vi "CalcCurrentThreshold.vi"(8 "Target Decimal Output":u8=1, 10 "Current Threshold":dbl=1000.0 format="%#_13g", 11 "Current of Output Pins":dbl[](array[numeric])) -> (0 "Threshold":dbl=1000.0 format="%#_13g", 3 "Target binary output":bool[](array[boolean]))   [LabVIEW 2018]
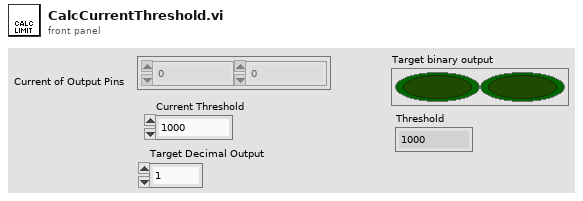
[diagram p1: front panel]
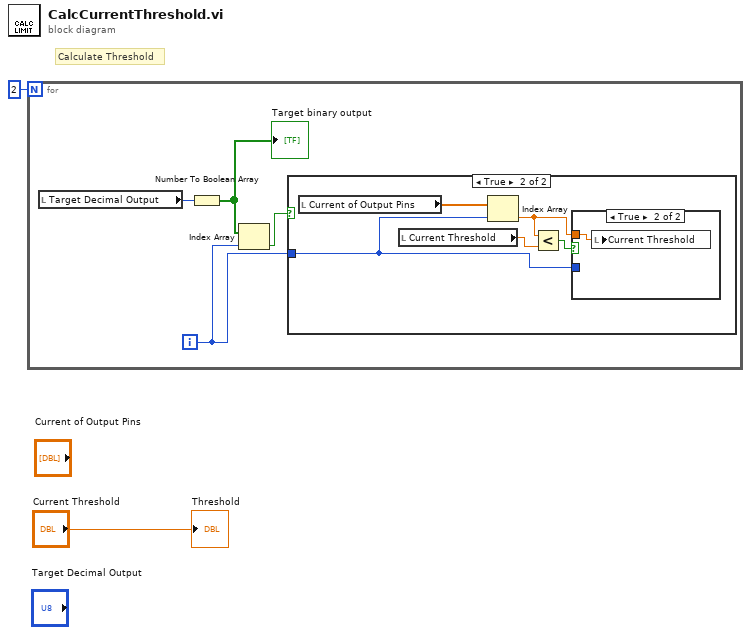
[diagram p0: block diagram]
diagram:
  # "Calculate Threshold"
  n1 = for {
    N: 2 -> [_]
    i -> [w4]
    n2 = local read "Target Decimal Output"() -> (w6:u8)
    n3 = Number To Boolean Array(number=w6) -> (Boolean array=w3:bool[])
    "Target binary output" <- w3
    n4 = Index Array(array=w3, index=w4) -> (element=w5:bool)
    n5 = case shown="True" w5 {
      tunnel: w4 -> [_ w11]
      frame False {
      }
      frame True {
        n6 = local read "Current of Output Pins"() -> (w9:dbl[])
        n7 = local read "Current Threshold"() -> (w7:dbl)
        n8 = Index Array(array=w9, index=w11) -> (element=w8:dbl)
        n9 = Less?(x=w8, y=w7) -> (x < y?=w10:bool)
        n10 = case shown="True" w10 {
          tunnel: w11 -> [_ _]
          tunnel: w8 -> [_ w12]
          frame False {
          }
          frame True {
            n11 = local write "Current Threshold"(w12) -> ()
          }
        }
      }
    }
  }
  "Threshold" <- "Current Threshold"
